vi "Count edges simple finite.vi"() -> ()   [LabVIEW 2023]
uses:
  <vilib>/Utility/error.llb/DialogType.ctl
  <vilib>/DAQmx/read.llb/DAQmx Read (Counter U32 1Chan 1Samp).vi
  <vilib>/DAQmx/create/channels.llb/DAQmx Create Channel (CI-Count Edges).vi
  <vilib>/DAQmx/miscellaneous.llb/DAQmx Fill In Error Info.vi
  <resource>/objmgr/daqmx.rc
panel:
  in  "milliseconds to wait":u32=3000
  in  "Active Edge":i32(ring)=10280 items=["Rising"=10280, "Falling"=10171]
  in  "Input Terminal":tag="/Dev1/PFI0"
  in  "Counter":tag="Dev1/ctr0"
  in  "Trigger Type":T1(tab)=enum."Digital Pause"
  in  "Edge":i32(ring)=10280 items=["Rising"=10280, "Falling"=10171]
  in  "Digital Trigger Source":tag
  in  "Pause When":i32(ring)=10214 items=["High"=10192, "Low"=10214]
  in  "Pause Trigger Source":tag="/Dev1/PFI9"
  in  "Count Reset Terminal":tag
  in  "Edge 2":i32(ring)=10280 items=["Rising"=10280, "Falling"=10171]
  out "Count":u32
  # "To configure and use a trigger or the count reset you must have the necessary tab selected above.  Not all hardware supports the above options--refer to your device documentation for more info."
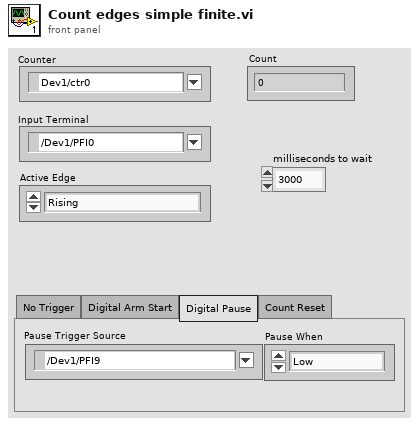
[diagram p1: front panel]
types:
  T1 = enum32{"No Trigger", "Digital Arm Start", "Digital Pause", "Count Reset"}
  T2 = typedef "DialogType.ctl" = u16
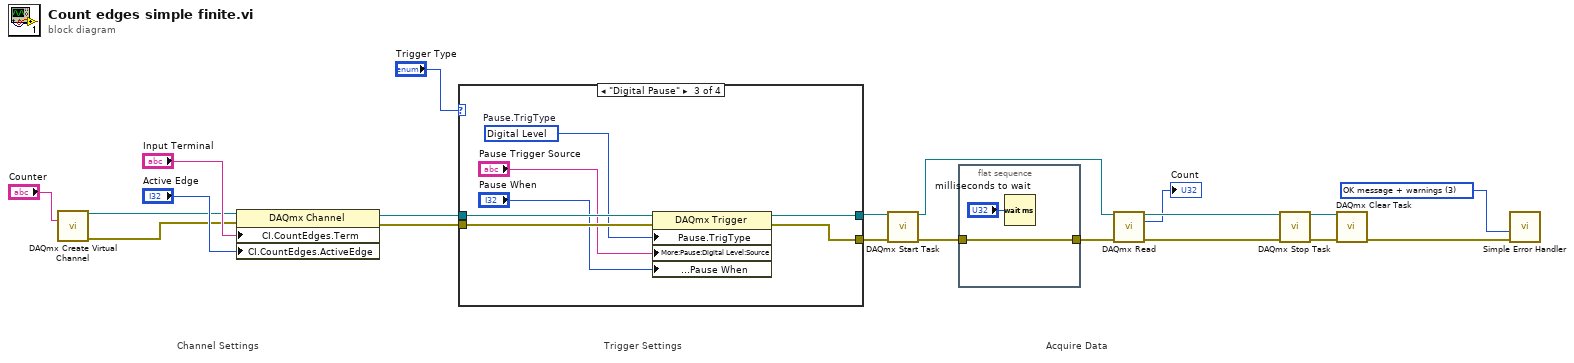
[diagram p0: block diagram]
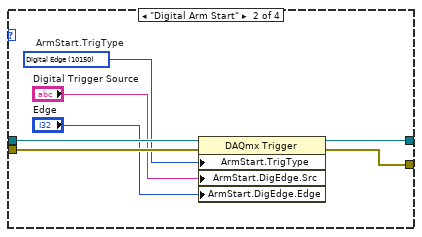
[diagram p3: hidden frame]
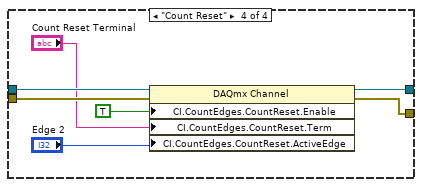
[diagram p4: hidden frame]
diagram:
  w5 = T2 3 items=["no dialog", "OK message", "continue or stop message", "OK message + warnings", "continue/stop + warnings"] ("type of dialog (OK msg:1)")
  # "Acquire Data"
  # "Trigger Settings"
  # "Channel Settings"
  n1 = call-poly <vilib>:"DAQmx Create Virtual Channel.vi"("counter"="Counter") -> ("task out"=w13:refnum<k21>, "error out"=w12:errorcluster)  [unwired: 13 in]
  n2 = property class="DAQmx Channel"(reference=w13, error in=w12, "CI.CountEdges.Term"="Input Terminal", "CI.CountEdges.ActiveEdge"="Active Edge") -> (reference out=w10:refnum<k21>, error out=w11:errorcluster)
  n3 = case shown="\"Digital Pause\"" "Trigger Type" {
    tunnel: w10 -> [w22 w29 w36 w43]
    tunnel: w11 -> [w21 w26 w33 w40]
    tunnel: [w22 w28 w35 w42] -> w18
    tunnel: [w21 w27 w34 w41] -> w17
    frame "No Trigger", Default {
    }
    frame "Digital Arm Start" {
      w23 = 10150 items=["Digital Edge"=10150, "None"=10230]  # ArmStart.TrigType
      n4 = property class="DAQmx Trigger"(reference=w29, error in=w26, "ArmStart.TrigType"=w23, "ArmStart.DigEdge.Src"="Digital Trigger Source", "ArmStart.DigEdge.Edge"="Edge") -> (reference out=w28:refnum<k21>, error out=w27:errorcluster)
    }
    frame "Digital Pause" {
      w32 = 10152 items=["Analog Level"=10101, "Analog Window"=10103, "Digital Level"=10152, "Digital Pattern"=10398, "None"=10230]  # Pause.TrigType
      n5 = property class="DAQmx Trigger"(reference=w36, error in=w33, "Pause.TrigType"=w32, "More:Pause:Digital Level:Source"="Pause Trigger Source", "More:Pause:Digital Level:Pause When"="Pause When") -> (reference out=w35:refnum<k21>, error out=w34:errorcluster)
    }
    frame "Count Reset" {
      n6 = property class="DAQmx Channel"(reference=w43, error in=w40, "CI.CountEdges.CountReset.Enable"=TRUE, "CI.CountEdges.CountReset.Term"="Count Reset Terminal", "CI.CountEdges.CountReset.ActiveEdge"="Edge 2") -> (reference out=w42:refnum<k21>, error out=w41:errorcluster)
    }
  }
  n7 = call <vilib>:"DAQmx Start Task.vi"("task/channels in"=w18, "error in"=w17) -> ("task out"=w1:refnum<k21>, "error out"=w3:errorcluster)  [unwired: 12 in]
  n8 = flat-sequence {
    tunnel: w3 -> [w45]
    tunnel: [w45] -> w2
    frame #0 {
      n9 = Wait (ms)(milliseconds to wait="milliseconds to wait") -> ()  [unwired: 1 out]
    }
  }
  n10 = call-poly <vilib>:"DAQmx Read.vi"("task/channels in"=w1, "error in"=w2) -> ("task out"=w9:refnum<k21>, "data"=→"Count":u32, "error out"=w8:errorcluster)  [unwired: 11 in]
  n11 = call <vilib>:"DAQmx Stop Task.vi"("task/channels in"=w9, "error in"=w8) -> ("task out"=w6:refnum<k21>, "error out"=w7:errorcluster)  [unwired: 12 in]
  n12 = call <vilib>:"DAQmx Clear Task.vi"("task in"=w6, "error in"=w7) -> ("error out"=w16:errorcluster)  [unwired: 13 in]
  n13 = call <vilib>:"Simple Error Handler.vi"("type of dialog (OK msg:1)"=w5, "error in (no error)"=w16) -> ()  [unwired: 3 in, 5 out]
